vi "Valid Name or Team.vi"(1 "Input Boolean":bool, 2 "Input String":string) -> (0 "Output String":string)   [LabVIEW 2011]
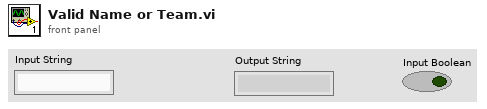
[diagram p1: front panel]
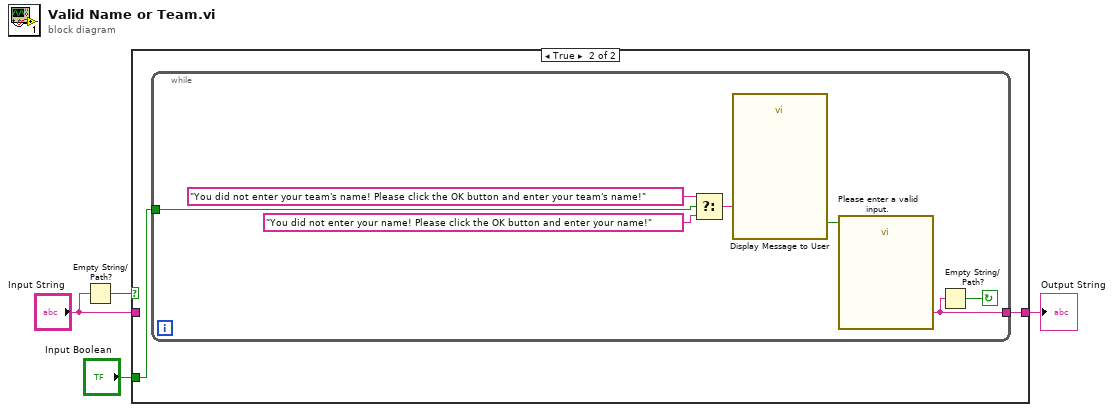
[diagram p0: block diagram]
diagram:
  n1 = Empty String/Path?(string/path="Input String") -> (empty?=w4:bool)
  n2 = case shown="True" w4 {
    tunnel: [w5 w6] -> w3
    tunnel: "Input String" -> [w5 _]
    tunnel: "Input Boolean" -> [_ w7]
    frame False {
    }
    frame True {
      n3 = while {
        tunnel: w7 -> [w12]
        tunnel: [w8] -> w6
        stop <- w9 continue-if-true
        n4 = Select(t="You did not enter your team's name! Please click the OK button and enter your team's name!", s=w12, f="You did not enter your name! Please click the OK button and enter your name!") -> (s? t:f=w11:string)
        n5 = call "Display Message to User"("Message"=w11) -> ("OK"=w10:bool)  [unwired: 9 in, 1 out]
        n6 = call "Please enter a valid input."("Enable"=w10) -> ("Input:"=w8:string)  [unwired: 16 in, 2 out]
        n7 = Empty String/Path?(string/path=w8) -> (empty?=w9:bool)
      }
    }
  }
  "Output String" <- w3
